vi "test31-MappingRelationshipByLocalRegistration_WIthoutSubscriberName_State.vi"(8 "error in (no error)":errorcluster, 11 "TestCase in":refnum<class "testcase-CSMBroadcast.lvclass">) -> (0 "error out":errorcluster, 3 "TestCase out":refnum<class "testcase-CSMBroadcast.lvclass">)   [LabVIEW 2017, in "testcase-CSMBroadcast.lvclass"]
uses:
  testcase-CSMBroadcast.lvclass
  47fe1622-87c8-40c1-b9cf-9bbb5cd90bb5.vi
  <vilib>/addons/_JKI Toolkits/VI Tester/TestCase.llb/TestCase.lvclass
  src/user.lib/_NEVSTOP/Communicable State Machine(CSM)/Communicable State Machine.lvlib
  CSM/CSM-Testcase.lvlib
  C:/Program Files (x86)/National Instruments/LabVIEW 2017/vi.lib/addons/_JKI Toolkits/VI Tester/TestCase.llb/TestCase.lvclass
panel:
  out "Loop Count":i32
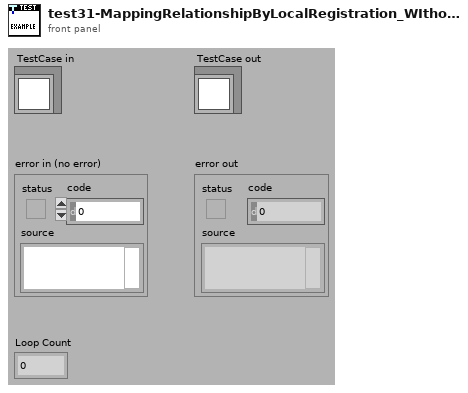
[diagram p1: front panel]
types:
  T1 = cluster{"Status":string, "Source CSM":string, "Target CSM":string, "Target API":string}[]
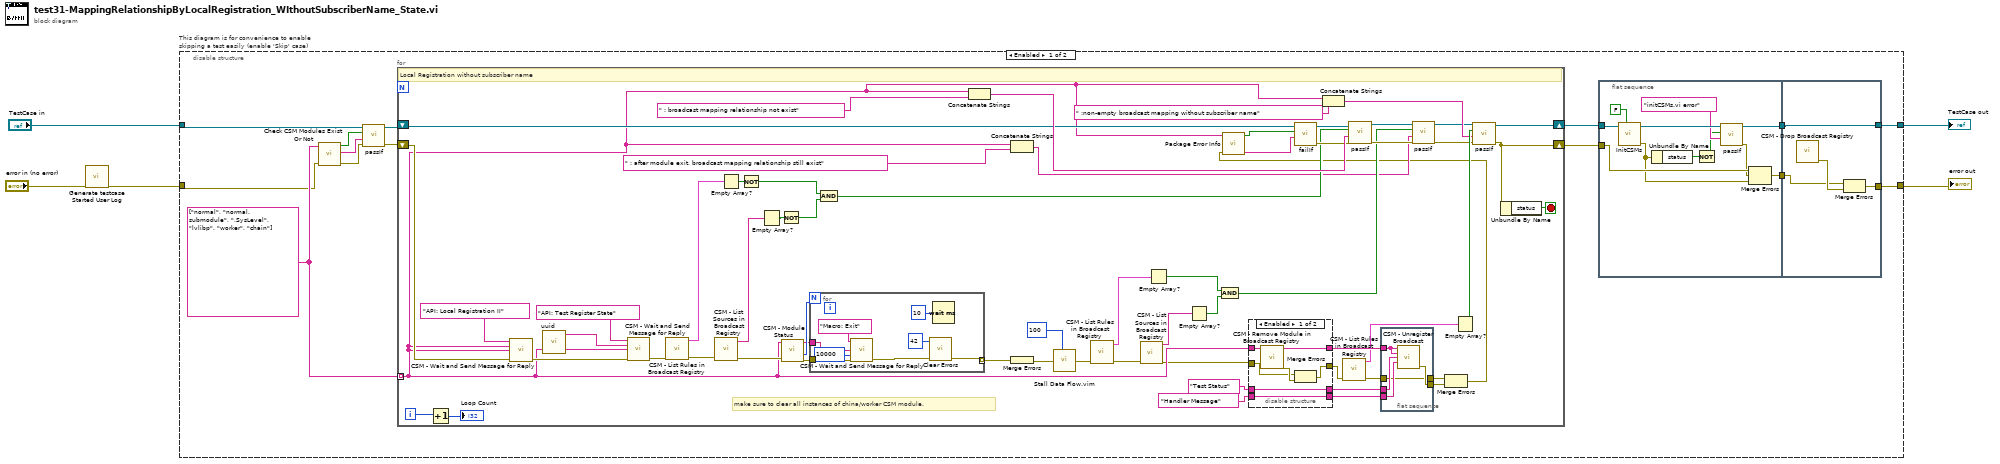
[diagram p0: block diagram]
diagram:
  n1 = call "Generate testcase Started User Log.vi"("Error In"="error in (no error)") -> ("error out"=w1:errorcluster)  [unwired: 10 in]
  n2 = disable-structure "This diagram is for convenience to enable skipping a test easily (enable 'Skip' case)" shown="Enabled" {
    disable-tunnel: "TestCase in" -> [w15 w124]
    disable-tunnel: [w9 w122] -> w2
    disable-tunnel: [w8 w123] -> w4
    disable-tunnel: w1 -> [w14 w121]
    frame Enabled {
      w16 = string[] ["normal", "normal.submodule", ".SysLevel", "lvlibp", "worker", "chain"]
      n3 = call "Check CSM Modules Exist Or Not.vi"("error in"=w14, "CSM names in"=w16) -> ("error out"=w17:errorcluster, "Debug string"=w18:string, "All Modules Exist?"=w19:bool)  [unwired: 7 in]
      n4 = call-dynamic "passIf.vi"("error in (no error)"=w17, "message (\"\")"=w18, "pass"=w19, "TestCase in"=w15) -> ("error out"=w6:errorcluster, "TestCase out"=w7:refnum<class "testcase-CSMBroadcast.lvclass">)  [unwired: 6 in]
      n5 = for {
        tunnel: w16 -> [w40] mode=indexing
        shift-right: [w80] -> w11
        shift-left: w7 -> [w63]
        shift-right: [w81] -> w10
        shift-left: w6 -> [w78]
        i -> [w87]
        stop <- w90 stop-if-true
        # "make sure to clear all instances of china/worker CSM module."
        # "Local Registration without subscriber name"
        n6 = Increment(x=w87) -> (x+1=→"Loop Count":i32)
        n7 = call "CSM - Wait and Send Message for Reply.vi"("State"="API: Local Registration II", "Arguments (\"\")"=w40, "Target Module"=w40, "Error In (No Error)"=w78) -> ("error out"=w95:errorcluster)  [unwired: 8 in, 3 out]
        n8 = call "uuid.vi"() -> ("UUID"=w93:string)  [unwired: 11 in]
        n9 = call "CSM - Wait and Send Message for Reply.vi"("State"="API: Test Register State", "Arguments (\"\")"=w93, "Target Module"=w40, "Error In (No Error)"=w95) -> ("error out"=w92:errorcluster)  [unwired: 8 in, 3 out]
        n10 = call "CSM - List Rules in Broadcast Registry.vi"("error in (no error)"=w92) -> ("error out"=w89:errorcluster, "Rule Entries"=w85:T1)  [unwired: 8 in, 1 out]
        n11 = call "CSM - List Sources in Broadcast Registry.vi"("error in (no error)"=w89) -> ("error out"=w75:errorcluster, "Broadcast Names"=w82:string[])  [unwired: 9 in]
        n12 = Empty Array?(array=w85) -> (empty?=w84:bool)
        n13 = Not(x=w84) -> (.not. x?=w61:bool)
        n14 = Empty Array?(array=w82) -> (empty?=w83:bool)
        n15 = Not(x=w83) -> (.not. x?=w60:bool)
        n16 = call "CSM - Module Status.vi"("Error In"=w75, "CSM Name"=w40) -> ("error out"=w74:errorcluster, "#Nodes"=w77:i32, "CSM Name (Dup)"=w76:string)  [unwired: 5 in, 2 out]
        n17 = for {
          N: w77 -> [_]
          tunnel: [w115] -> w91 mode=indexing
          tunnel: w76 -> [w119]
          tunnel: w74 -> [w118]
          n18 = call "CSM - Wait and Send Message for Reply.vi"("State"="Macro: Exit", "Target Module"=w119, "Wait (5000ms)"=10000, "Error In (No Error)"=w118) -> ("error out"=w116:errorcluster)  [unwired: 8 in, 3 out]
          n19 = call <vilib>:"Clear Errors.vi"("error in (no error)"=w116, "specific error code to clear (0: all)"=42) -> ("error out"=w115:errorcluster)  [unwired: 4 in, 1 out]
          n20 = Wait (ms)(milliseconds to wait=u32 10) -> ()  [unwired: 1 out]
        }
        n21 = And(x=w61, y=w60) -> (x .and. y?=w59:bool)
        n22 = Concatenate Strings(w40, " : broadcast mapping relationship not exist" ("string")) -> (w70:string)
        n23 = Concatenate Strings(w40, " : after module exit, broadcast mapping relationship still exist" ("string")) -> (w48:string)
        n24 = Merge Errors(w91) -> (w69:errorcluster)
        n25 = call "Stall Data Flow.vim"("value in"=w69, "milliseconds to wait"=u32 100) -> ("value out"=w68:errorcluster)  [unwired: 1 out]
        n26 = call "CSM - List Rules in Broadcast Registry.vi"("error in (no error)"=w68) -> ("error out"=w88:errorcluster, "Rule Entries"=w54:T1)  [unwired: 8 in, 1 out]
        n27 = call "CSM - List Sources in Broadcast Registry.vi"("error in (no error)"=w88) -> ("error out"=w39:errorcluster, "Broadcast Names"=w53:string[])  [unwired: 9 in]
        n28 = Empty Array?(array=w54) -> (empty?=w52:bool)
        n29 = Empty Array?(array=w53) -> (empty?=w51:bool)
        n30 = And(x=w52, y=w51) -> (x .and. y?=w50:bool)
        n31 = disable-structure shown="Enabled" {
          disable-tunnel: w39 -> [w102 w111]
          disable-tunnel: [w106 w111] -> w46
          disable-tunnel: w40 -> [w107 w112]
          disable-tunnel: "Test Status" ("Status") -> [w104 w110]
          disable-tunnel: "Handler Message" ("Response Message (If \"\", Same as Source Message)") -> [w103 w109]
          disable-tunnel: [w105 w112] -> w47
          disable-tunnel: [w104 w110] -> w45
          disable-tunnel: [w103 w109] -> w44
          frame Enabled {
            n32 = call "CSM - Remove Module in Broadcast Registry.vi"("CSM Name"=w107) -> ("CSM Name (Dup)"=w105:string, "error out"=w108:errorcluster)  [unwired: 13 in]
            n33 = Merge Errors(w102, w108) -> (w106:errorcluster)
          }
          frame Disabled {
          }
        }
        n34 = Concatenate Strings(w40, " :non-empty broadcast mapping without subscriber name" ("string")) -> (w71:string)
        n35 = call "CSM - List Rules in Broadcast Registry.vi"("error in (no error)"=w46) -> ("error out"=w42:errorcluster, "Rule Entries"=w35:T1)  [unwired: 8 in, 1 out]
        n36 = flat-sequence {
          tunnel: w47 -> [w101]
          tunnel: w45 -> [w100]
          tunnel: w44 -> [w99]
          tunnel: [w98] -> w43
          tunnel: w42 -> [w97]
          tunnel: [w97] -> w41
          frame #0 {
            n37 = call "CSM - Unregister Broadcast.vi"("CSM Name(Empty for Broadcast Event)"=w101, "Source CSM Name (* as Default)"=w101, "Trigger"=w100, "API (\"*\" as Default)"=w99) -> ("error out"=w98:errorcluster)  [unwired: 10 in, 1 out]
          }
        }
        n38 = Merge Errors(w41, w43) -> (w38:errorcluster)
        n39 = call "Package Error Info.vi"("error in"=w38, "String in"=w40) -> ("packed error info out"=w66:string, "error status"=w65:bool)  [unwired: 8 in]
        n40 = call-dynamic "failIf.vi"("message (\"\")"=w66, "fail"=w65, "TestCase in"=w63) -> ("error out"=w64:errorcluster, "TestCase out"=w62:refnum<class "testcase-CSMBroadcast.lvclass">)  [unwired: 7 in]
        n41 = call-dynamic "passIf.vi"("error in (no error)"=w64, "message (\"\")"=w70, "pass"=w59, "TestCase in"=w62) -> ("error out"=w56:errorcluster, "TestCase out"=w58:refnum<class "testcase-CSMBroadcast.lvclass">)  [unwired: 6 in]
        n42 = call-dynamic "passIf.vi"("error in (no error)"=w56, "message (\"\")"=w48, "pass"=w50, "TestCase in"=w58) -> ("error out"=w55:errorcluster, "TestCase out"=w57:refnum<class "testcase-CSMBroadcast.lvclass">)  [unwired: 6 in]
        n43 = Empty Array?(array=w35) -> (empty?=w79:bool)
        n44 = call-dynamic "passIf.vi"("error in (no error)"=w55, "message (\"\")"=w71, "pass"=w79, "TestCase in"=w57) -> ("error out"=w81:errorcluster, "TestCase out"=w80:refnum<class "testcase-CSMBroadcast.lvclass">)  [unwired: 6 in]
        n45 = Unbundle By Name(w81) -> ("status"=w90:bool)
      }
      n46 = flat-sequence {
        tunnel: w11 -> [w30]
        tunnel: [w27] -> w13
        tunnel: w10 -> [w24]
        tunnel: [w21] -> w12
        tunnel: w13 -> [w33]
        tunnel: [w33] -> w9
        tunnel: [w32] -> w8
        tunnel: w12 -> [w31]
        frame #0 {
          n47 = call "InitCSMs.vi"("Enable building lvlibp?"=FALSE, "testcase-CSMStatus in"=w30) -> ("error out"=w22:errorcluster, "testcase-CSMStatus out"=w28:refnum<class "testcase-CSMBroadcast.lvclass">)  [unwired: 8 in]
          n48 = Unbundle By Name(w22) -> ("status"=w26:bool)
          n49 = Not(x=w26) -> (.not. x?=w20:bool)
          n50 = call-dynamic "passIf.vi"("message (\"\")"="initCSMs.vi error" ("message (\"\")"), "pass"=w20, "TestCase in"=w28) -> ("error out"=w23:errorcluster, "TestCase out"=w27:refnum<class "testcase-CSMBroadcast.lvclass">)  [unwired: 7 in]
          n51 = Merge Errors(w24, w23, w22) -> (w21:errorcluster)
        }
        frame #1 {
          n52 = call "CSM - Drop Broadcast Registry.vi"() -> ("error out"=w34:errorcluster)  [unwired: 15 in]
          n53 = Merge Errors(w31, w34) -> (w32:errorcluster)
        }
      }
    }
    frame Disabled {
      # "skip test result while test is under development"
      n54 = call <vilib>:"skip.vi"("error in (no error)"=w121, "TestCase in"=w124) -> ("error out"=w123:errorcluster, "TestCase out"=w122:refnum<class "testcase-CSMBroadcast.lvclass">)  [unwired: 8 in]
    }
  }
  "error out" <- w4
  "TestCase out" <- w2
